vi "内置函数VI Tree.vi"   [LabVIEW 2013]
uses:
  <resource>/importtools/Common/Event/NISAST Event.lvclass
  <vilib>/UserTags/UserTags.lvlib
  <vilib>/CommandQueue/Command Queue.lvlib
  <vilib>/DotNET/AssemblyVisualizationTool/DotNETAssemblyVisualizer.lvlib
  <vilib>/Utility/lvfile.llb/NI_FileType.lvlib
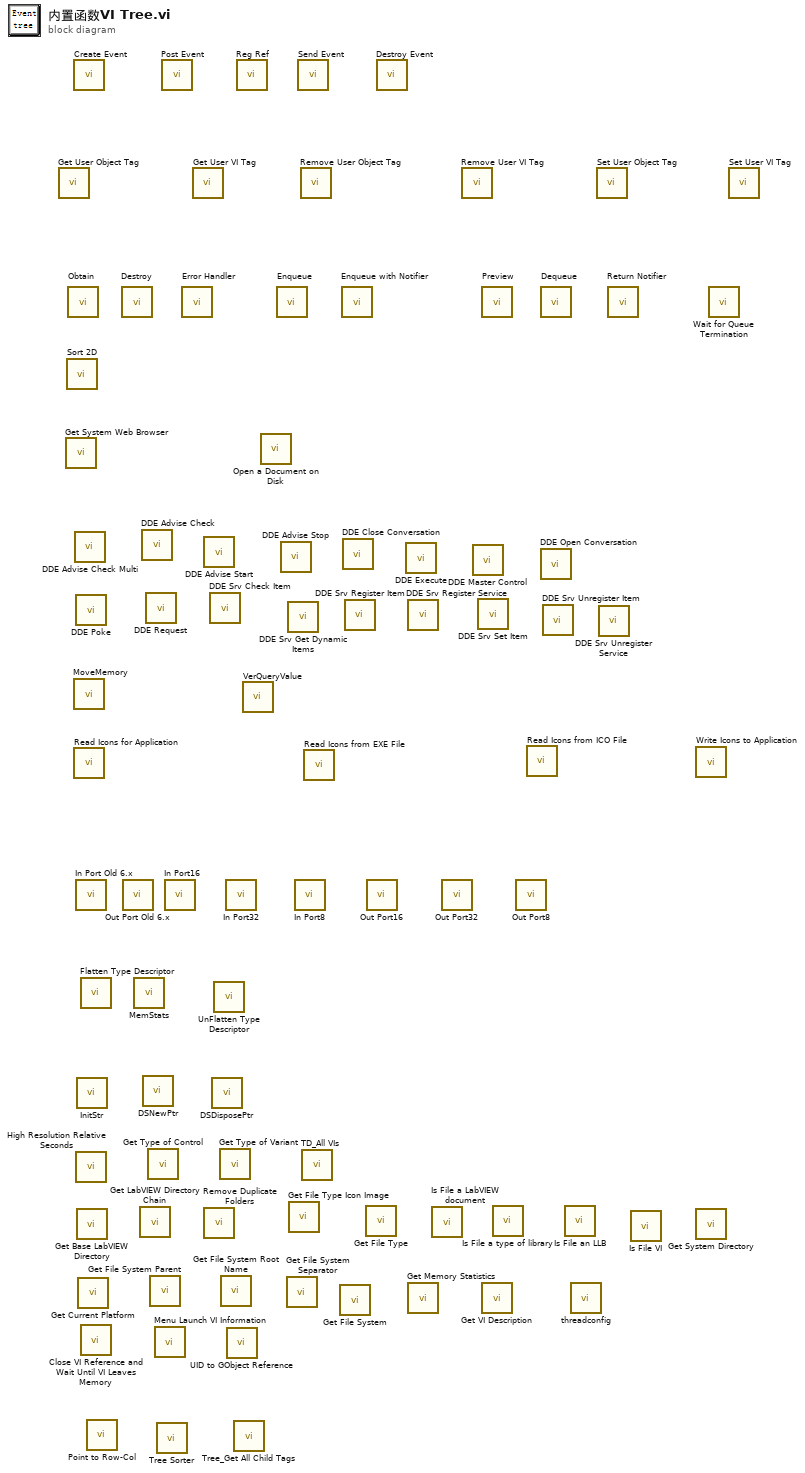
[diagram p0: block diagram]
diagram:
  n1 = call <vilib>:"Get User Object Tag.vi"() -> ()  [unwired: 8 in, 4 out]
  n2 = call <vilib>:"Get System Web Browser.vi"() -> ()  [unwired: 6 in, 2 out]
  n3 = call <vilib>:"Sort 2D.vi"() -> ()  [unwired: 4 in, 1 out]
  n4 = call <vilib>:"Obtain.vi"() -> ()  [unwired: 9 in, 3 out]
  n5 = call-dynamic "Create Event.vi"() -> ()  [unwired: 9 in, 3 out]
  n6 = call <vilib>:"MoveMemory.vi"() -> ()  [unwired: 10 in, 2 out]
  n7 = call <vilib>:"Read Icons for Application.vi"() -> ()  [unwired: 8 in, 4 out]
  n8 = call <vilib>:"DDE Advise Check Multi.vi"() -> ()  [unwired: 8 in, 2 out]
  n9 = call <vilib>:"DDE Poke.vi"() -> ()  [unwired: 8 in, 2 out]
  n10 = call <vilib>:"In Port Old 6.x.vi"() -> ()  [unwired: 2 in, 1 out]
  n11 = call <vilib>:"High Resolution Relative Seconds.vi"() -> ()  [unwired: 1 out]
  n12 = call <vilib>:"InitStr.vi"() -> ()  [unwired: 10 in, 2 out]
  n13 = call <vilib>:"Get Base LabVIEW Directory.vi"() -> ()  [unwired: 8 in, 4 out]
  n14 = call <vilib>:"Get Current Platform.vi"() -> ()  [unwired: 7 in, 1 out]
  n15 = call <vilib>:"Flatten Type Descriptor.vi"() -> ()  [unwired: 5 in, 1 out]
  n16 = call <vilib>:"Close VI Reference and Wait Until VI Leaves Memory.vi"() -> ()  [unwired: 11 in, 1 out]
  n17 = call <vilib>:"Point to Row-Col.vi"() -> ()  [unwired: 6 in, 6 out]
  n18 = call <vilib>:"Destroy.vi"() -> ()  [unwired: 9 in, 3 out]
  n19 = call <vilib>:"Out Port Old 6.x.vi"() -> ()  [unwired: 3 in]
  n20 = call <vilib>:"MemStats.vi"() -> ()  [unwired: 5 in, 3 out]
  n21 = call <vilib>:"Get LabVIEW Directory Chain.vi"() -> ()  [unwired: 8 in, 4 out]
  n22 = call <vilib>:"DDE Advise Check.vi"() -> ()  [unwired: 6 in, 4 out]
  n23 = call <vilib>:"DSNewPtr.vi"() -> ()  [unwired: 10 in, 2 out]
  n24 = call <vilib>:"DDE Request.vi"() -> ()  [unwired: 7 in, 3 out]
  n25 = call <vilib>:"Get Type of Control.vi"() -> ()  [unwired: 9 in, 3 out]
  n26 = call <vilib>:"Get File System Parent.vi"() -> ()  [unwired: 1 out]
  n27 = call <vilib>:"Menu Launch VI Information.vi"() -> ()  [unwired: 9 in, 3 out]
  n28 = call <vilib>:"Tree Sorter.vi"() -> ()  [unwired: 9 in, 1 out]
  n29 = call-dynamic "Post Event.vi"() -> ()  [unwired: 10 in, 2 out]
  n30 = call <vilib>:"In Port16.vi"() -> ()  [unwired: 8 in, 2 out]
  n31 = call <vilib>:"Error Handler.vi"() -> ()  [unwired: 10 in, 2 out]
  n32 = call <vilib>:"Get User VI Tag.vi"() -> ()  [unwired: 8 in, 4 out]
  n33 = call <vilib>:"DDE Advise Start.vi"() -> ()  [unwired: 8 in, 2 out]
  n34 = call <vilib>:"Remove Duplicate Folders.vi"() -> ()  [unwired: 11 in, 1 out]
  n35 = call <vilib>:"DDE Srv Check Item.vi"() -> ()  [unwired: 6 in, 4 out]
  n36 = call <vilib>:"DSDisposePtr.vi"() -> ()  [unwired: 11 in, 1 out]
  n37 = call <vilib>:"UnFlatten Type Descriptor.vi"() -> ()  [unwired: 5 in, 1 out]
  n38 = call <vilib>:"Get Type of Variant.vi"() -> ()  [unwired: 10 in, 2 out]
  n39 = call <vilib>:"Get File System Root Name.vi"() -> ()  [unwired: 1 out]
  n40 = call <vilib>:"In Port32.vi"() -> ()  [unwired: 8 in, 2 out]
  n41 = call <vilib>:"UID to GObject Reference.vi"() -> ()  [unwired: 9 in, 3 out]
  n42 = call <vilib>:"Tree_Get All Child Tags.vi"() -> ()  [unwired: 9 in, 3 out]
  n43 = call-dynamic "Reg Ref.vi"() -> ()  [unwired: 9 in, 3 out]
  n44 = call <vilib>:"VerQueryValue.vi"() -> ()  [unwired: 9 in, 3 out]
  n45 = call <vilib>:"Open a Document on Disk.vi"() -> ()  [unwired: 7 in, 1 out]
  n46 = call <vilib>:"Enqueue.vi"() -> ()  [unwired: 9 in, 3 out]
  n47 = call <vilib>:"DDE Advise Stop.vi"() -> ()  [unwired: 8 in, 2 out]
  n48 = call <vilib>:"Get File System Separator.vi"() -> ()  [unwired: 1 out]
  n49 = call <vilib>:"DDE Srv Get Dynamic Items.vi"() -> ()  [unwired: 8 in, 2 out]
  n50 = call <vilib>:"Get File Type Icon Image.vi"() -> ()  [unwired: 10 in, 2 out]
  n51 = call <vilib>:"In Port8.vi"() -> ()  [unwired: 8 in, 2 out]
  n52 = call-dynamic "Send Event.vi"() -> ()  [unwired: 9 in, 3 out]
  n53 = call <vilib>:"Remove User Object Tag.vi"() -> ()  [unwired: 9 in, 3 out]
  n54 = call <vilib>:"TD_All VIs.vi"() -> ()  [unwired: 1 in]
  n55 = call <vilib>:"Read Icons from EXE File.vi"() -> ()  [unwired: 8 in, 4 out]
  n56 = call <vilib>:"Get File System.vi"() -> ()  [unwired: 1 out]
  n57 = call <vilib>:"Enqueue with Notifier.vi"() -> ()  [unwired: 9 in, 3 out]
  n58 = call <vilib>:"DDE Close Conversation.vi"() -> ()  [unwired: 9 in, 1 out]
  n59 = call <vilib>:"DDE Srv Register Item.vi"() -> ()  [unwired: 8 in, 2 out]
  n60 = call <vilib>:"Get File Type.vi"() -> ()  [unwired: 9 in, 3 out]
  n61 = call <vilib>:"Out Port16.vi"() -> ()  [unwired: 9 in, 1 out]
  n62 = call-dynamic "Destroy Event.vi"() -> ()  [unwired: 10 in, 2 out]
  n63 = call <vilib>:"DDE Execute.vi"() -> ()  [unwired: 8 in, 2 out]
  n64 = call <vilib>:"DDE Srv Register Service.vi"() -> ()  [unwired: 8 in, 2 out]
  n65 = call <vilib>:"Get Memory Statistics.vi"() -> ()  [unwired: 3 in, 3 out]
  n66 = call <vilib>:"Is File a LabVIEW document.vi"() -> ()  [unwired: 10 in, 2 out]
  n67 = call <vilib>:"Out Port32.vi"() -> ()  [unwired: 9 in, 1 out]
  n68 = call <vilib>:"Remove User VI Tag.vi"() -> ()  [unwired: 9 in, 3 out]
  n69 = call <vilib>:"DDE Master Control.vi"() -> ()  [unwired: 5 in, 5 out]
  n70 = call <vilib>:"DDE Srv Set Item.vi"() -> ()  [unwired: 8 in, 2 out]
  n71 = call <vilib>:"Preview.vi"() -> ()  [unwired: 7 in, 5 out]
  n72 = call <vilib>:"Get VI Description.vi"() -> ()  [unwired: 10 in, 2 out]
  n73 = call <vilib>:"Is File a type of library.vi"() -> ()  [unwired: 10 in, 2 out]
  n74 = call <vilib>:"Out Port8.vi"() -> ()  [unwired: 9 in, 1 out]
  n75 = call <vilib>:"Read Icons from ICO File.vi"() -> ()  [unwired: 7 in, 5 out]
  n76 = call <vilib>:"Dequeue.vi"() -> ()  [unwired: 7 in, 5 out]
  n77 = call <vilib>:"DDE Open Conversation.vi"() -> ()  [unwired: 8 in, 2 out]
  n78 = call <vilib>:"DDE Srv Unregister Item.vi"() -> ()  [unwired: 8 in, 2 out]
  n79 = call <vilib>:"Is File an LLB.vi"() -> ()  [unwired: 10 in, 2 out]
  n80 = call <vilib>:"threadconfig.vi"() -> ()  [unwired: 1 out]
  n81 = call <vilib>:"Set User Object Tag.vi"() -> ()  [unwired: 9 in, 3 out]
  n82 = call <vilib>:"DDE Srv Unregister Service.vi"() -> ()  [unwired: 9 in, 1 out]
  n83 = call <vilib>:"Return Notifier.vi"() -> ()  [unwired: 11 in, 1 out]
  n84 = call <vilib>:"Is File VI.vi"() -> ()  [unwired: 9 in, 3 out]
  n85 = call <vilib>:"Write Icons to Application.vi"() -> ()  [unwired: 10 in, 2 out]
  n86 = call <vilib>:"Get System Directory.vi"() -> ()  [unwired: 11 in, 1 out]
  n87 = call <vilib>:"Wait for Queue Termination.vi"() -> ()  [unwired: 11 in, 1 out]
  n88 = call <vilib>:"Set User VI Tag.vi"() -> ()  [unwired: 9 in, 3 out]
